vi "myRIO_BRig_RT_dataExp_Cue1Param_AudioLed_Probability_NS.vi"() -> (2 "output_Cue1Param_AudioLed_Probability_NS":i32)   [LabVIEW 2014]
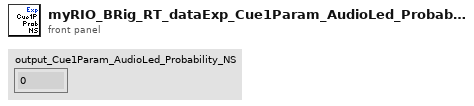
[diagram p1: front panel]
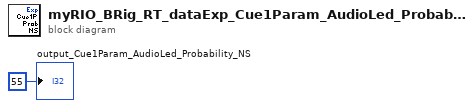
[diagram p0: block diagram]
diagram:
  "output_Cue1Param_AudioLed_Probability_NS" <- 55 ("output_iBlock")
